vi "addDocument[]Element.vi"(7 "Name":string, 8 "error in (no error)":errorcluster, 9 "Value":refnum<class "tBSONDocument.lvclass">[](array[class]), 10 "Replace? (false)":bool, 11 "tBSONDocument in":refnum<class "tBSONDocument.lvclass">) -> (0 "error out":errorcluster, 3 "tBSONDocument out":refnum<class "tBSONDocument.lvclass">)   [LabVIEW 2013, in "BSON.lvlib" / "tBSONDocument.lvclass"]
doc: "Adds an array of BSON Documents as an element in a BSON document."
uses:
  tBSONDocument.lvclass
  tBSONElement/tBSONElement.lvclass
  BSONElements/tBSONDocumentElement/tBSONDocumentElement.lvclass
  BSONElements/tBSONDocumentElement/setValue.vi
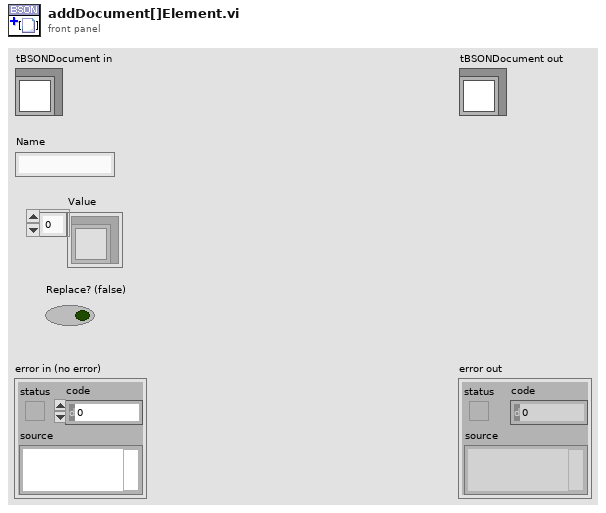
[diagram p1: front panel]
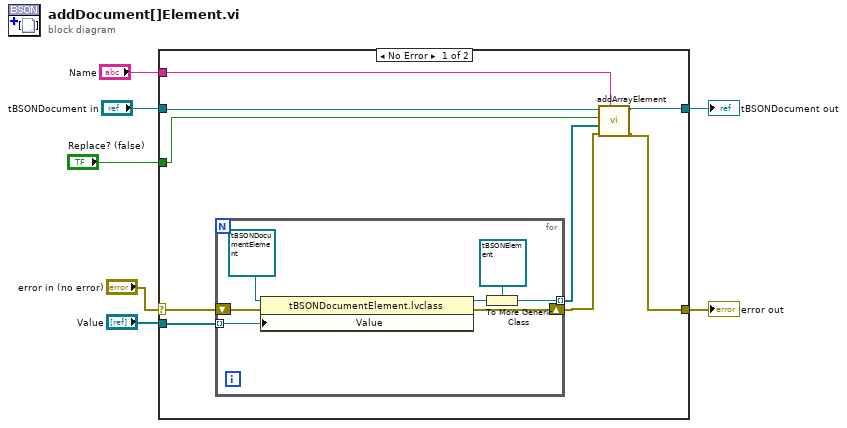
[diagram p0: block diagram]
diagram:
  n1 = case shown="No Error" "error in (no error)" {
    selector: "error in (no error)" -> [w16 w25]
    tunnel: [w12 w25] -> w2
    tunnel: [w11 w24] -> w7
    tunnel: "tBSONDocument in" -> [w15 w24]
    tunnel: "Name" -> [w10 _]
    tunnel: "Value" -> [w9 _]
    tunnel: "Replace? (false)" -> [w8 _]
    frame No Error {
      n2 = for {
        tunnel: w9 -> [w18] mode=indexing
        shift-right: [w22] -> w14
        shift-left: w16 -> [w23]
        tunnel: [w19] -> w13 mode=indexing
        n3 = property class="tBSONDocumentElement.lvclass"(reference=refnum<class "tBSONDocumentElement.lvclass"> refnum ("BSON.lvlib:tBSONDocumentElement.lvclass"), error in=w23, "Value"=w18) -> (reference out=w21:refnum<class "tBSONDocumentElement.lvclass">, error out=w22:errorcluster)
        n4 = To More Generic Class(target class=refnum<class "tBSONElement.lvclass"> refnum ("BSON.lvlib:tBSONElement.lvclass"), reference=w21) -> (generic class reference=w19:refnum<class "tBSONElement.lvclass">)
      }
      n5 = call "addArrayElement.vi"("Name"=w10, "error in (no error)"=w14, "Value"=w13, "Replace? (false)"=w8, "tBSONDocument in"=w15) -> ("error out"=w12:errorcluster, "tBSONDocument out"=w11:refnum<class "tBSONDocument.lvclass">)  [unwired: 5 in]
    }
    frame Error {
    }
  }
  "error out" <- w2
  "tBSONDocument out" <- w7
